vi "ReturnToStartPosition_Original.vi"(8 "Desired offset from switch":dbl=-500.0 format="%.2f", 9 "DO Task":refnum<k21>="BlueSimple_DO") -> ()   [LabVIEW 2010]
uses:
  Controls/Bits to Write.ctl
panel:
  out "String":string
  out "sine offset size":string
  out "concatenated string":string
  out "Must move":dbl
  out "Current Position":dbl format="%.2f"
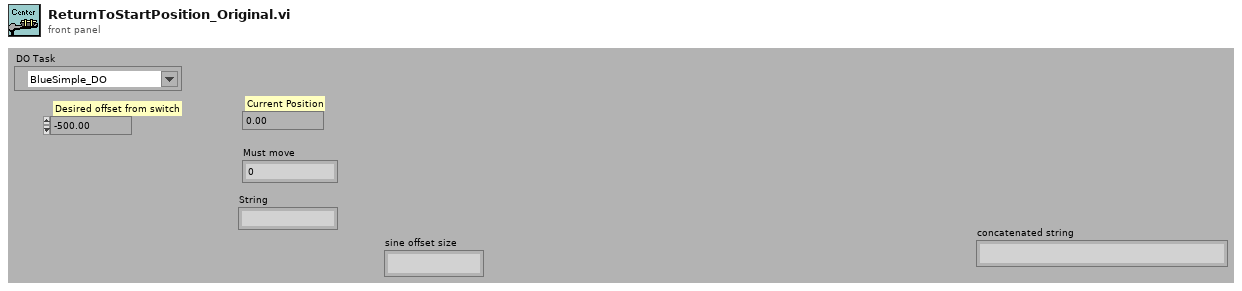
[diagram p1: front panel]
types:
  T1 = typedef "Bits to Write.ctl" = enum16{"LED 1 on", "LED 1 off", "LED 2 on", "LED 2 off", "LED 3 on", "LED 3 off", "LED 4 on", "LED 4 off", "All LEDs on", "All LEDs off", "In trial on", "In trial off", "Buzzer on", "Buzzer off", "Reward on", "Reward off", "Target number", "Trial type preQ on", "Trial type preQ off", "Error on", "Error off", "Trial number", "DBS on", "DBS off", "Sine on", "Sine off", "All Bits On", "All Bits Off", "Init", "Specify mask/pattern"}
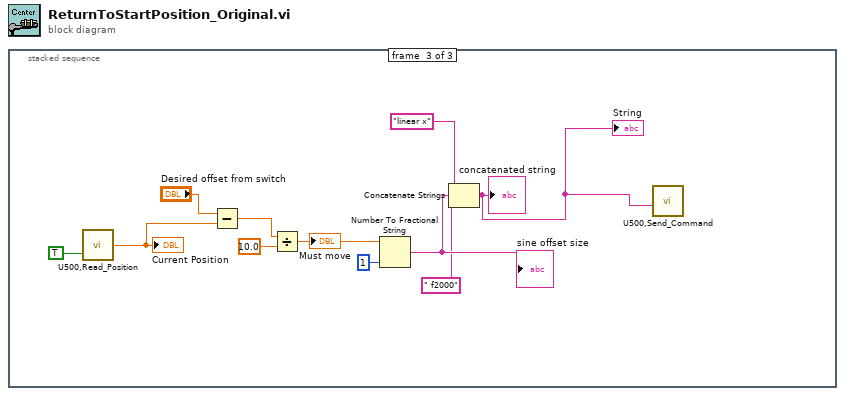
[diagram p0: block diagram]
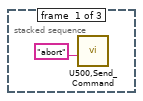
[diagram p2: hidden frame]
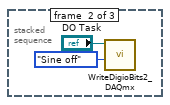
[diagram p3: hidden frame]
diagram:
  n1 = stacked-sequence {
    frame #0 {
      n2 = call "U500,Send_Command.vi"("Command String"="abort") -> ()  [unwired: 9 in, 2 out]
    }
    frame #1 {
      n3 = call "WriteDigioBits2_DAQmx.vi"("Bits to write"=Bits_to_Write."Sine off", "DO Task"="DO Task") -> ()  [unwired: 9 in, 1 out]
    }
    frame #2 {
      n4 = call "U500,Read_Position.vi"("Auto Update"=TRUE) -> ("Position"=w12:dbl)  [unwired: 1 in]
      "Current Position" <- w12
      n5 = Subtract(x="Desired offset from switch", y=w12) -> (x-y=w11:dbl)
      n6 = Divide(x=w11, y=10.0) -> (x/y=w5:dbl)
      "Must move" <- w5
      n7 = Number To Fractional String(number=w5, precision (6)=i16 1) -> (F-format string=w7:string)  [unwired: 2 in]
      "sine offset size" <- w7
      n8 = Concatenate Strings("linear x" ("Command String"), w7, " f2000" ("string")) -> (w4:string)
      "concatenated string" <- w4
      "String" <- w4
      n9 = call "U500,Send_Command.vi"("Command String"=w4) -> ()  [unwired: 9 in, 2 out]
    }
  }
